vi "Get Tweets Old.vi"(8 "error in":errorcluster, 9 "Tweets to Read (10)":i32=10 min=0 max=200 step=1, 10 "Screen Name (Empty)":string, 11 "Twitter Handle In":T2={"OAuth Credentials"={"Consumer Key"="", "Signature Method"=enum."HMAC-SHA1", "Token"="", "Version"="", "Token Secret"="", "Consumer Secret"=""}, "since ID"="", "max ID"="", "Screen Name"=""}) -> (0 "error out":errorcluster, 1 "Actual Num of Tweets Read":i32, 2 "Old Tweets Read":T1[](array[typedef]), 3 "Twitter Handle Out":T2={"OAuth Credentials"={"Consumer Key"="", "Signature Method"=enum."HMAC-SHA1", "Token"="", "Version"="", "Token Secret"="", "Consumer Secret"=""}, "since ID"="", "max ID"="", "Screen Name"=""}, 5 "Time Stamp of Oldest Tweet":timestamp)   [LabVIEW 2011, in "i3-twitter.lvlib"]
doc: "Get old tweets for the screen name. If no screen name is provided, tweets for the authenticating user are returned."
uses:
  i3-twitter.lvlib
  Controls/Twitter Handle.ctl
  i3-oauth/Controls/OAuth Credentials.ctl
  i3-oauth/Controls/Signature Method.ctl
  Controls/Tweet.ctl
  i3-oauth/Controls/HTTP Method.ctl
  i3-json/JSON Parsing/Get Array Value at Index Files/Get Array Value at Index - Object.vi
  i3-json/JSON Parsing/Get Object Parameter Files/Get Object Parameter - String.vi
  i3-json/JSON Parsing/Get Object Parameter Files/Get Object Parameter - Object.vi
  i3-oauth/i3-oauth.lvlib
  <vilib>/httpClient/LabVIEWHTTPClient.lvlib
  i3-json/i3-json.lvlib
panel:
  out "headers":string
  out "body":string
  out "Full URL":string
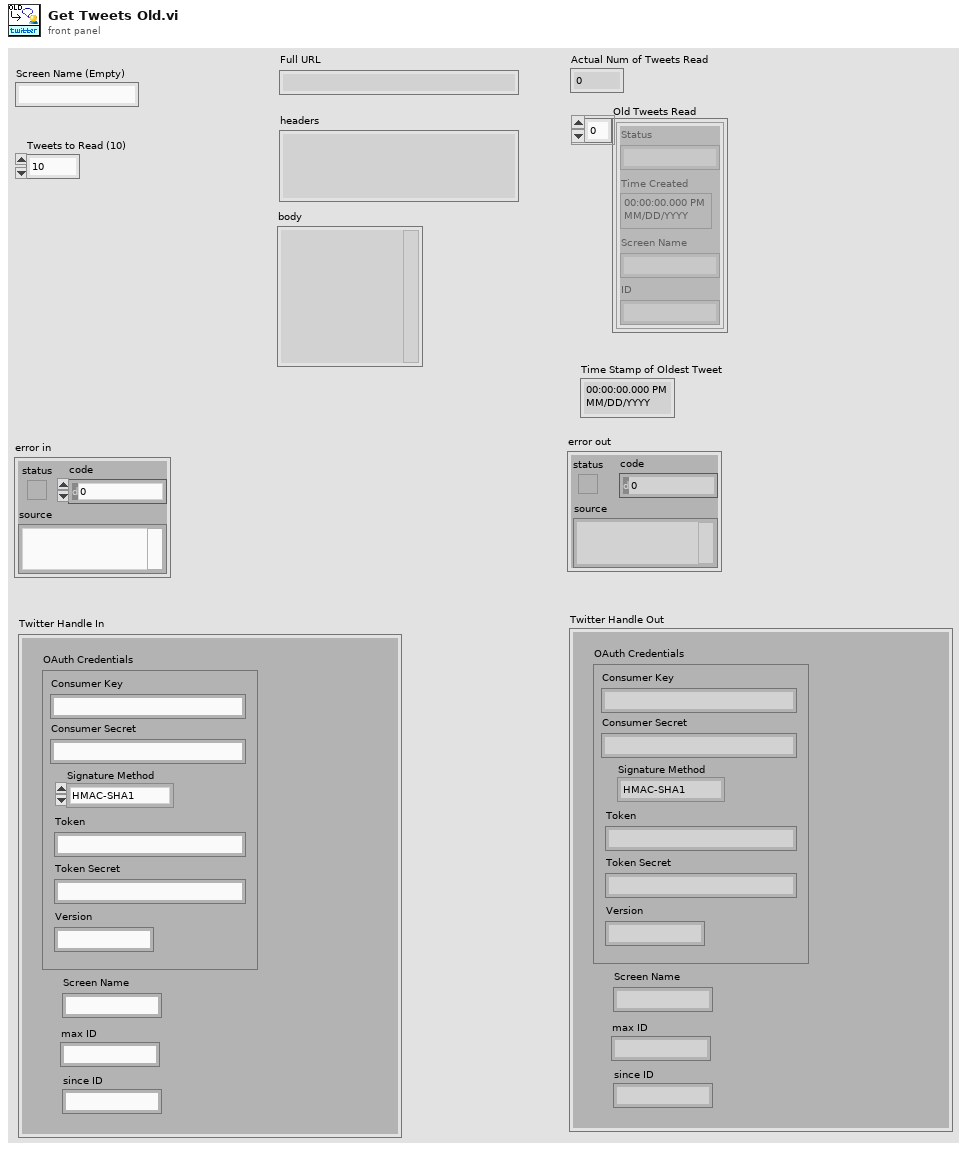
[diagram p1: front panel]
types:
  T1 = typedef "i3-twitter.lvlib/Tweet.ctl" = cluster{"Status":string, "Time Created":timestamp, "Screen Name":string, "ID":string}
  T2 = typedef "i3-twitter.lvlib/Twitter Handle.ctl" = cluster{"OAuth Credentials":T3, "since ID":string, "max ID":string, "Screen Name":string}
  T3 = typedef "i3-oauth.lvlib/OAuth Credentials.ctl" = cluster{"Consumer Key":string, "Signature Method":T4, "Token":string, "Version":string, "Token Secret":string, "Consumer Secret":string}
  T4 = typedef "i3-oauth.lvlib/Signature Method.ctl" = enum16{"HMAC-MD5", "HMAC-SHA1", "HMAC-SHA224", "HMAC-SHA256", "HMAC-SHA384", "HMAC-SHA512"}
  T5 = typedef "i3-oauth.lvlib/HTTP Method.ctl" = enum16{"GET", "POST", "PUT", "DELETE"}
  T6 = typedef "i3-oauth.lvlib/key-value-pairs.ctl" = cluster{"key":string, "value":string}
  T7 = typedef "LabVIEWHTTPClient.lvlib/ClientHandle.ctl" = refnum<k1>
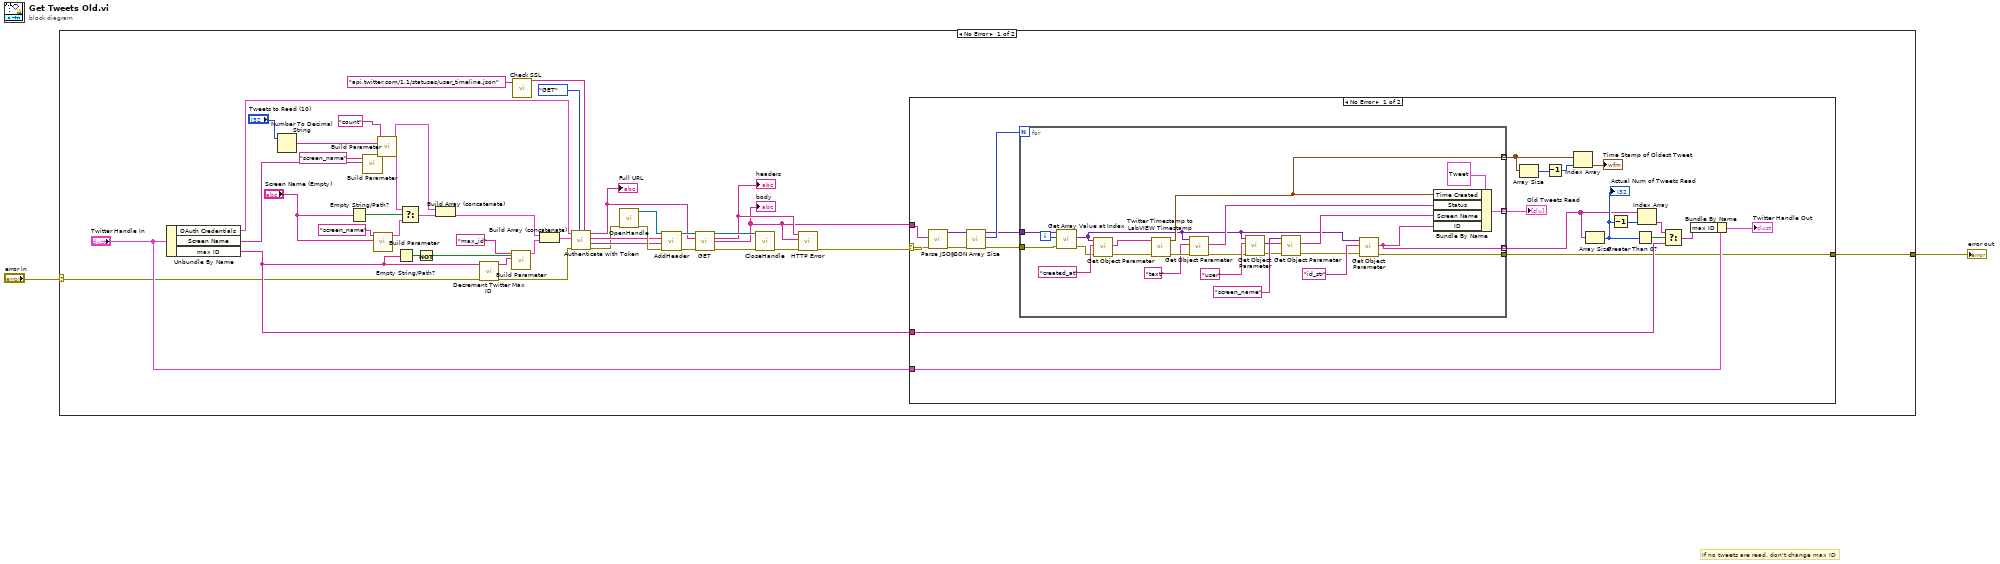
[diagram p0: block diagram]
diagram:
  # "If no tweets are read, don't change max ID"
  n1 = case shown="No Error" "error in" {
    selector: "error in" -> [w7 w92]
    tunnel: [w11 w92] -> w2
    frame No Error {
      n2 = Unbundle By Name("Twitter Handle In") -> ("OAuth Credentials"=w3:T3, "Screen Name"=w9:string, "max ID"=w8:string)
      n3 = Number To Decimal String(number="Tweets to Read (10)") -> (decimal integer string=w33:string)  [unwired: 1 in]
      n4 = Empty String/Path?(string/path="Screen Name (Empty)") -> (empty?=w20:bool)
      n5 = call "Build Parameter.vi"("Value"=w9, "Key"="screen_name") -> ("Parameter Array"=w18:T6[])  [unwired: 9 in]
      n6 = call "Build Parameter.vi"("Value"="Screen Name (Empty)", "Key"="screen_name") -> ("Parameter Array"=w17:T6[])  [unwired: 9 in]
      n7 = call "Build Parameter.vi"("Value"=w33, "Key"="count") -> ("Parameter Array"=w31:T6[])  [unwired: 9 in]
      n8 = Empty String/Path?(string/path=w8) -> (empty?=w27:bool)
      n9 = Select(t=w18, s=w20, f=w17) -> (s? t:f=w19:T6[])
      n10 = Not(x=w27) -> (.not. x?=w23:bool)
      n11 = Build Array (concatenate)(w31, w19) -> (w30:T6[])
      n12 = call "Decrement Twitter Max ID.vi"("error in (no error)"=w7, "ID In"=w8) -> ("error out"=w16:errorcluster, "ID Out"=w24:string)  [unwired: 8 in]
      n13 = call "Build Parameter.vi"("Return Parameter? (T)"=w23, "Value"=w24, "Key"="max_id") -> ("Parameter Array"=w26:T6[])  [unwired: 8 in]
      n14 = call "Check SSL.vi"("Input URL"="api.twitter.com/1.1/statuses/user_timeline.json" ("Base URL")) -> ("Output URL"=w4:string)  [unwired: 8 in]
      n15 = Build Array (concatenate)(w30, w26) -> (w29:T6[])
      n16 = call "Authenticate with Token.vi"("Base URL"=w4, "HTTP Method"=HTTP_Method."GET", "error in (no error)"=w16, "URL Parameters"=w29, "OAuth Credentials"=w3) -> ("error out"=w28:errorcluster, "Header Value"=w37:string, "Header Parameter"=w38:string, "Full URL"=w36:string)  [unwired: 2 in, 1 out]
      "Full URL" <- w36
      n17 = call <vilib>:"OpenHandle.vi"("error in (no error)"=w28) -> ("client handle out"=w44:T7, "error out"=w43:errorcluster)  [unwired: 13 in]
      n18 = call <vilib>:"AddHeader.vi"("client handle"=w44, "header"=w38, "value"=w37, "error in (no error)"=w43) -> ("client handle out"=w42:T7, "error out"=w41:errorcluster)  [unwired: 10 in]
      n19 = call <vilib>:"GET.vi"("client handle"=w42, "url"=w36, "error in (no error)"=w41) -> ("client handle out"=w40:T7, "headers"=w15:string, "body"=w10:string, "error out"=w39:errorcluster)  [unwired: 9 in]
      "body" <- w10
      "headers" <- w15
      n20 = call <vilib>:"CloseHandle.vi"("client handle"=w40, "error in (no error)"=w39) -> ("error out"=w14:errorcluster)  [unwired: 13 in]
      n21 = call "HTTP Error.vi"("error in (no error)"=w14, "Body"=w10, "Header"=w15) -> ("error out"=w12:errorcluster)  [unwired: 6 in, 2 out]
      n22 = case shown="No Error" w12 {
        selector: w12 -> [w52 w91]
        tunnel: w8 -> [w55 _]
        tunnel: "Twitter Handle In" -> [w54 _]
        tunnel: [w51 w91] -> w11
        tunnel: w10 -> [w50 _]
        frame No Error {
          n23 = call "Parse JSON.vi"("error in (no error)"=w52, "JSON String"=w50) -> ("error out"=w64:errorcluster, "JSON Tree"=w65:variant)  [unwired: 6 in, 2 out]
          n24 = call "JSON Array Size.vi"("error in (no error)"=w64, "JSON Tree In (JSON Array)"=w65) -> ("error out"=w63:errorcluster, "Array Size"=w66:i32, "JSON Tree Passthrough (JSON Array)"=w56:variant)  [unwired: 7 in]
          n25 = for {
            N: w66 -> [_]
            tunnel: [w79] -> w48 mode=indexing
            tunnel: w63 -> [w75]
            tunnel: [w80] -> w62 mode=indexing
            tunnel: [w83] -> w51
            tunnel: w56 -> [w74]
            tunnel: [w73] -> w47 mode=indexing
            i -> [w85]
            n26 = call-poly "Get Array Value at Index.vi"("error in (no error)"=w75, "Index"=w85, "JSON Tree In (JSON Array)"=w74) -> ("error out"=w82:errorcluster, "JSON Object"=w71:variant)  [unwired: 5 in, 2 out]
            n27 = call-poly "Get Object Parameter.vi"("error in (no error)"=w82, "Parameter Name"="created_at", "JSON Tree In (JSON Object)"=w71) -> ("error out"=w69:errorcluster, "String Value"=w68:string)  [unwired: 5 in, 2 out]
            n28 = call "Twitter Timestamp to LabVIEW Timestamp.vi"("error in"=w69, "Twitter Time Stamp"=w68) -> ("error out"=w78:errorcluster, "LabVIEW Time Stamp"=w73:timestamp)  [unwired: 6 in]
            n29 = call-poly "Get Object Parameter.vi"("error in (no error)"=w78, "Parameter Name"="text", "JSON Tree In (JSON Object)"=w71) -> ("error out"=w67:errorcluster, "String Value"=w76:string)  [unwired: 5 in, 2 out]
            n30 = call-poly "Get Object Parameter.vi"("error in (no error)"=w67, "Parameter Name"="user", "JSON Tree In (JSON Object)"=w71) -> ("error out"=w81:errorcluster, "JSON Object"=w70:variant)  [unwired: 5 in, 2 out]
            n31 = call-poly "Get Object Parameter.vi"("error in (no error)"=w81, "Parameter Name"="screen_name", "JSON Tree In (JSON Object)"=w70) -> ("error out"=w77:errorcluster, "String Value"=w88:string)  [unwired: 5 in, 2 out]
            n32 = call-poly "Get Object Parameter.vi"("error in (no error)"=w77, "Parameter Name"="id_str", "JSON Tree In (JSON Object)"=w71) -> ("error out"=w83:errorcluster, "String Value"=w79:string)  [unwired: 5 in, 2 out]
            n33 = Bundle By Name(cluster=T1 {"Status"="", "Time Created"=timestamp(0 s since 1904-01-01), "Screen Name"="", "ID"=""}, "Time Created"=w73, "Status"=w76, "Screen Name"=w88, "ID"=w79) -> (w80:T1)
          }
          "Old Tweets Read" <- w62
          n34 = Array Size(array=w47) -> (size(s)=w46:i32)
          n35 = Decrement(x=w46) -> (x-1=w45:i32)
          n36 = Index Array(array=w47, index=w45) -> (element=→"Time Stamp of Oldest Tweet":timestamp)
          n37 = Array Size(array=w48) -> (size(s)=w59:i32)
          "Actual Num of Tweets Read" <- w59
          n38 = Decrement(x=w59) -> (x-1=w61:i32)
          n39 = Greater Than 0?(x=w59) -> (x > 0?=w60:bool)
          n40 = Index Array(array=w48, index=w61) -> (element=w58:string)
          n41 = Select(t=w58, s=w60, f=w55) -> (s? t:f=w57:string)
          n42 = Bundle By Name(cluster=w54, "max ID"=w57) -> (→"Twitter Handle Out":T2)
        }
        frame Error {
        }
      }
    }
    frame Error {
    }
  }
  "error out" <- w2
